vi "Initialize.vi"(7 "Timeout (30 msec)":u32=30, 8 "error in (no error)":errorcluster, 9 "Force Baud Rate (True)":bool=TRUE, 10 "Baud rate (57600 bps)":T1=34 items=["1,000,000 bps"=1, "500,000 bps"=3, "400,000 bps"=4, "250,000 bps"=7, "200,000 bps"=9, "115200 bps"=16, "57600 bps"=34, "19200 bps"=103, "9600 bps"=207], 11 "VISA resource name":refnum<visa-resource-name>) -> (0 "error out":errorcluster, 3 "VISA resource name out":refnum<visa-resource-name>)   [LabVIEW 2016]
doc: "Establishes communication with the instrument and optionally performs an instrument identification query and/or an instrument reset. It also places the instrument in a default state needed for other instrument driver operations. Therefore, call this VI before calling other instrument driver VIs for this instrument. Generally, you need to call the Initialize VI only once at the beginning of an application."
uses:
  Motor Operation/Low Level/Baud Setting.ctl
  <vilib>/Instr/_visa.llb/VISA Configure Serial Port (Instr).vi
  Dynamixel Motor.lvlib
panel:
  # "(c) 2011-2012  National Instruments.  ALL RIGHTS RESERVED."
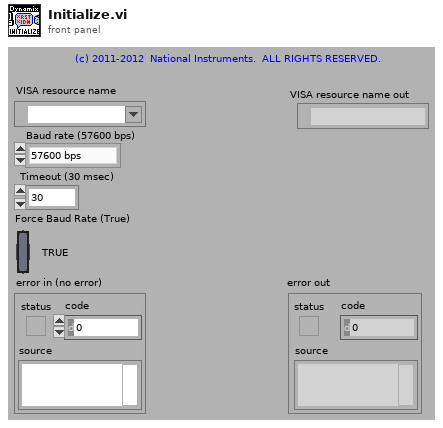
[diagram p1: front panel]
types:
  T1 = typedef "Dynamixel Motor.lvlib/Baud Setting.ctl" = u8
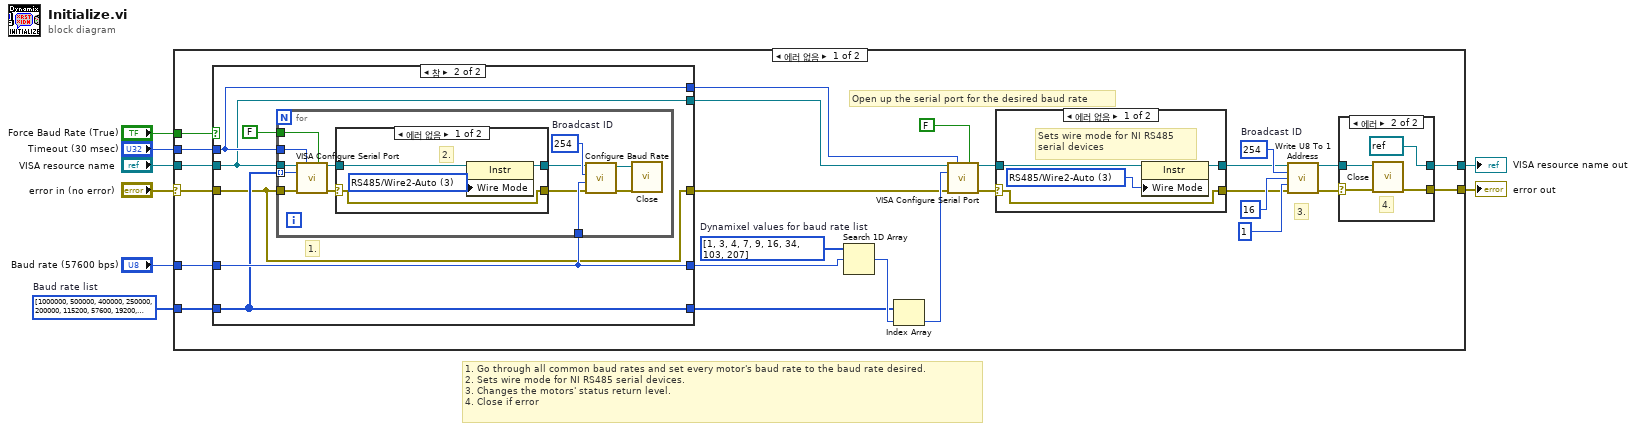
[diagram p0: block diagram]
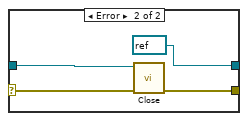
[diagram p2: hidden frame]
diagram:
  w2 = u32[] [1000000, 500000, 400000, 250000, 200000, 115200, 57600, 19200, 9600]  # Baud rate list
  # "1. Go through all common baud rates and set every motor's baud rate to the baud rate desired.\n2. Sets wire mode for NI RS485 serial devices.\n3. Changes the motors' status return level.\n4. Close if error"
  n1 = case shown="에러 없음" "error in (no error)" {
    selector: "error in (no error)" -> [w9 w80]
    tunnel: [w34 w79] -> w8
    tunnel: [w33 w80] -> w7
    tunnel: "VISA resource name" -> [w24 w79]
    tunnel: "Timeout (30 msec)" -> [w23 _]
    tunnel: "Baud rate (57600 bps)" -> [w22 _]
    tunnel: "Force Baud Rate (True)" -> [w25 _]
    tunnel: w2 -> [w21 _]
    frame No Error {
      w19 = u8[] [1, 3, 4, 7, 9, 16, 34, 103, 207]  # Dynamixel values for baud rate list
      w32 = u8 254  # Broadcast ID
      # "Open up the serial port for the desired baud rate"
      # "3."
      n2 = case shown="참" w25 {
        tunnel: w24 -> [w43 w48]
        tunnel: w9 -> [w44 w49]
        tunnel: w23 -> [w45 w50]
        tunnel: w22 -> [w47 w52]
        tunnel: w21 -> [w46 w51]
        tunnel: [w47 w52] -> w14
        tunnel: [w46 w51] -> w13
        tunnel: [w45 w50] -> w12
        tunnel: [w44 w49] -> w11
        tunnel: [w43 w48] -> w10
        frame False {
        }
        frame True {
          # "1."
          n3 = for {
            tunnel: w48 -> [w66]
            tunnel: w49 -> [w65]
            tunnel: w50 -> [w64]
            tunnel: FALSE ("Enable Termination\nChar (T)") -> [w63]
            tunnel: w51 -> [w62] mode=indexing
            tunnel: w52 -> [w58]
            w61 = u8 254  # Broadcast ID
            n4 = call-poly "VISA Configure Serial Port"("VISA resource name"=w66, "timeout (10sec)"=w64, "Enable Termination\nChar (T)"=w63, "baud rate (9600)"=w62, "error in (no error)"=w65) -> ("VISA resource name out"=w57:refnum<visa-resource-name>, "error out"=w56:errorcluster)  [unwired: 9 in]
            n5 = case shown="에러 없음" w56 {
              selector: w56 -> [w67 w71]
              tunnel: w57 -> [w70 w72]
              tunnel: [w68 w72] -> w55
              tunnel: [w67 w71] -> w54
              frame No Error {
                w69 = i16 3 items=["Unknown"=-1, "RS485/Wire4"=0, "RS485/Wire2-EchoDTR"=1, "RS485/Wire2-CtrlDTR"=2, "RS485/Wire2-Auto"=3, "RS232/DTE"=128, "RS232/DCE"=129, "RS232/AUTO"=130] ("Serial Settings:Wire Mode")
                # "2."
                n6 = property class="Instr"(reference=w70, "Wire Mode"=w69) -> (reference out=w68:refnum<visa-resource-name>)  [unwired: 1 in, 1 out]
              }
              frame Error {
              }
            }
            n7 = call "Configure Baud Rate.vi"("error in (no error)"=w54, "Baud rate (57600 bps)"=w58, "Motor ID (0)"=w61, "VISA resource name"=w55) -> ("error out"=w59:errorcluster, "VISA resource name out"=w60:refnum<visa-resource-name>)  [unwired: 6 in]
            n8 = call "Close.vi"("error in (no error)"=w59, "VISA resource name"=w60) -> ()  [unwired: 9 in, 1 out]
          }
        }
      }
      n9 = Search 1D Array(1D array=w19, element=w14) -> (index of element=w18:i32)  [unwired: 1 in]
      n10 = Index Array(array=w13, index=w18) -> (element=w17:u32)
      n11 = call-poly "VISA Configure Serial Port"("VISA resource name"=w10, "timeout (10sec)"=w12, "Enable Termination\nChar (T)"=FALSE ("Enable Termination\nChar (T)"), "baud rate (9600)"=w17, "error in (no error)"=w11) -> ("VISA resource name out"=w16:refnum<visa-resource-name>, "error out"=w15:errorcluster)  [unwired: 9 in]
      n12 = case shown="에러 없음" w15 {
        selector: w15 -> [w38 w40]
        tunnel: w16 -> [w35 w42]
        tunnel: [w36 refnum<visa-resource-name> refnum ("VISA resource name out")] -> w27
        tunnel: [w38 w39] -> w26
        frame No Error {
          w37 = i16 3 items=["Unknown"=-1, "RS485/Wire4"=0, "RS485/Wire2-EchoDTR"=1, "RS485/Wire2-CtrlDTR"=2, "RS485/Wire2-Auto"=3, "RS232/DTE"=128, "RS232/DCE"=129, "RS232/AUTO"=130] ("Serial Settings:Wire Mode")
          # "Sets wire mode for NI RS485\nserial devices"
          n13 = property class="Instr"(reference=w35, "Wire Mode"=w37) -> (reference out=w36:refnum<visa-resource-name>)  [unwired: 1 in, 1 out]
        }
        frame Error {
          n14 = call "Close.vi"("error in (no error)"=w40, "VISA resource name"=w42) -> ("error out"=w39:errorcluster)  [unwired: 9 in]
        }
      }
      n15 = call "Write U8 To 1 Address.vi"("VISA resource name"=w27, "Motor ID (0)"=w32, "Address number (0)"=u8 16, "Parameter (0)"=u8 1, "error in (no error)"=w26) -> ("VISA resource name out"=w29:refnum<visa-resource-name>, "error out"=w30:errorcluster)  [unwired: 9 in]
      n16 = case shown="에러" w30 {
        selector: w30 -> [w74 w77]
        tunnel: [w73 refnum<visa-resource-name> refnum ("VISA resource name out")] -> w34
        tunnel: [w74 w78] -> w33
        tunnel: w29 -> [w73 w75]
        frame No Error {
        }
        frame Error {
          # "4."
          n17 = call "Close.vi"("error in (no error)"=w77, "VISA resource name"=w75) -> ("error out"=w78:errorcluster)  [unwired: 9 in]
        }
      }
    }
    frame Error {
    }
  }
  "VISA resource name out" <- w8
  "error out" <- w7
